vi "GPX_position_test.vi"() -> ()   [LabVIEW 2020]
panel:
  out "pos distance [m]":dbl
  out "acceleration graph":cluster{timestamp[], dbl[]}[](graph)
  out "gps mean speed":dbl format="%0.2f"
  out "distance [m]":dbl
  in  "shift [s]":dbl
  in  "Shift":bool
  out "delta t [s]":dbl
  in  "stop":bool
  in  "reset":bool
  in  "binary path (use dialog)":path
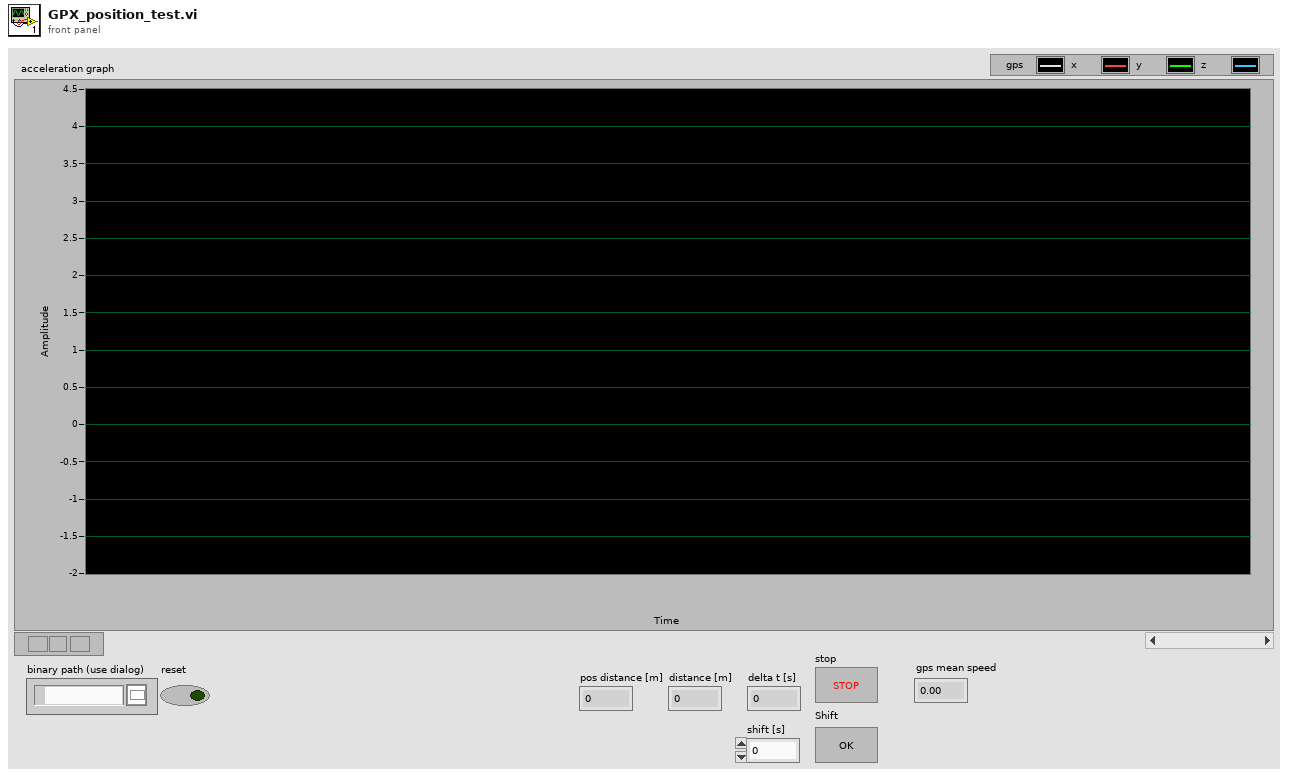
[diagram p1: front panel]
types:
  T1 = typedef "control_time_informations.ctl" = cluster{"starting time":timestamp, "ending time":timestamp, "dt[s]":dbl, "sampling rate [Hz]":dbl, "length":dbl}
  T2 = typedef "control_all_in_one_package.ctl" = cluster{"memory structure":T3, "actigraph settings":T4, "time informations":T1, "measurement data":T5}
  T3 = typedef "control_memory_structure.ctl" = cluster{"length of metadata [byte]":i32, "length of page [byte]":i32, "length of measurement data on page [byte]":i32, "length of dataset [byte]":i32}
  T4 = typedef "control_measurement_settings.ctl" = cluster{"sampling frequency [Hz]":dbl, "measurement interval [± g]":i32, "high precision?":bool, "number of pages":i32, "rate code":i32, "range code":i32, "id":i32}
  T5 = typedef "control_measurement_data.ctl" = cluster{"number of samples per axis":i32, "timestamp array":dbl[], "offset array":dbl[], "x, y, z axis data":waveform(dbl)[], "normalised magnitude of acceleartion vectors":waveform(dbl), "calibration coefficients":T6, "statistics":T7, "battery voltage":waveform(dbl), "magnitude of acceleartion vectors":waveform(dbl)}
  T6 = typedef "control_calibration_coefficients.ctl" = cluster{"Sx":dbl, "Ox":dbl, "Sy":dbl, "Oy":dbl, "Sz":dbl, "Oz":dbl}
  T7 = typedef "control_statistics.ctl" = cluster{"mean of x axis acceleration":dbl, "standard devation of x axis acceleration":dbl, "mean of y axis acceleration":dbl, "standard devation of y axis acceleration":dbl, "mean of z axis acceleration":dbl, "standard devation of z axis acceleration":dbl, "mean of normalised magnitude of acceleration":dbl, "standard devation of normalised magnitude of acceleration":dbl}
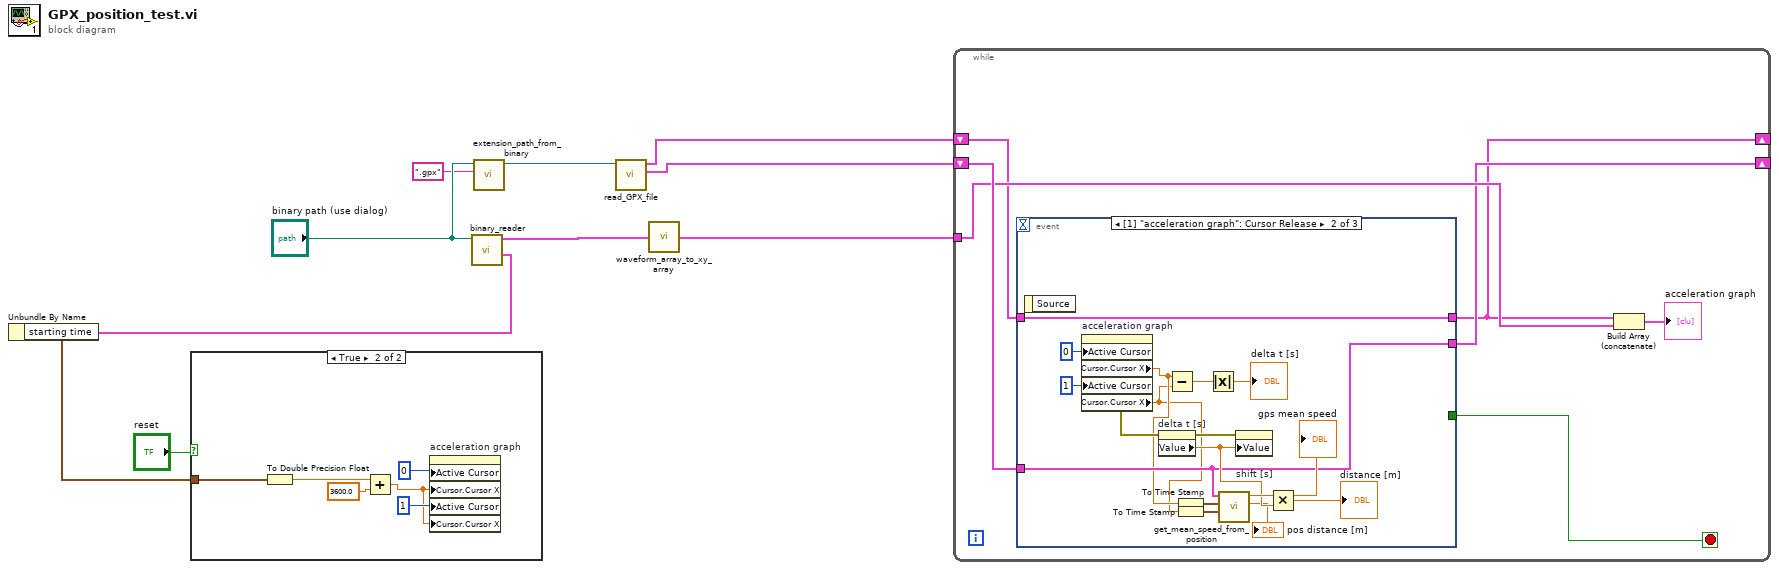
[diagram p0: block diagram]
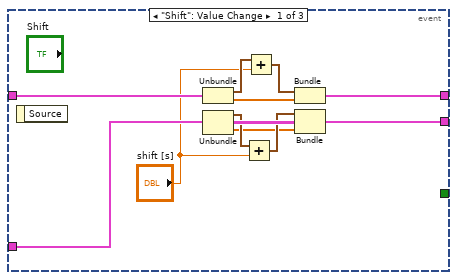
[diagram p2: hidden frame]
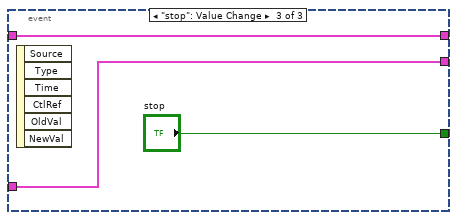
[diagram p3: hidden frame]
diagram:
  n1 = call "binary_reader.vi"("path to binary file"="binary path (use dialog)") -> ("time informations"=w9:T1, "all in one package"=w7:T2)  [unwired: 7 in, 1 out]
  n2 = Unbundle By Name(w9) -> ("starting time"=w8:timestamp)
  n3 = case shown="True" "reset" {
    tunnel: w8 -> [_ w14]
    frame False {
    }
    frame True {
      n4 = To Double Precision Float(number=w14) -> (double precision float=w15:dbl)
      n5 = Add(x=w15, y=3600.0) -> (x+y=w11:dbl)
      n6 = property on="acceleration graph" class="XYGraph (strict)"("Active Cursor"=u32 0, "Cursor.Cursor X"=w11, "Active Cursor"=u32 1, "Cursor.Cursor X"=w11) -> ()  [unwired: 2 in, 2 out]
    }
  }
  n7 = call "extension_path_from_binary.vi"("extension"=".gpx", "path to binary file"="binary path (use dialog)") -> ("path to file"=w2:path)  [unwired: 9 in]
  n8 = call "read_GPX_file.vi"("GPX File Path"=w2) -> ("lat/lon position"=w5:cluster{timestamp[], dbl[], dbl[]}, "XY Speed data"=w4:cluster{timestamp[], dbl[]})  [unwired: 3 in, 2 out]
  n9 = call "waveform_array_to_xy_array.vi"("waveform array"=w7) -> ("XY array"=w6:cluster{timestamp[], "Y":dbl[]}[])
  n10 = while {
    shift-right: [w19] -> _
    shift-left: w5 -> [w22]
    tunnel: w6 -> [w20]
    shift-right: [w17] -> _
    shift-left: w4 -> [w18]
    stop <- w23 stop-if-true
    n11 = event shown="[1] \"acceleration graph\": Cursor Release" {
      selector: _ -> [_ _ _]
      dyn-events: _ -> [_ _ _]
      timeout: _ -> [_ _ _]
      tunnel: [_ _ "stop"] -> w23
      tunnel: [w31 w42 w53] -> w19
      tunnel: w22 -> [w35 w42 w53]
      tunnel: w18 -> [w29 w37 w52]
      tunnel: [w24 w37 w52] -> w17
      event "Shift": Value Change {
        n12 = event-data() -> ()  [unwired: 1 in, 1 out]
        n13 = Unbundle(w29) -> (w28:timestamp[], w25:dbl[])
        n14 = Unbundle(w35) -> (w34:timestamp[], w32:dbl[], w30:dbl[])
        n15 = Add(x=w34, y="shift [s]") -> (x+y=w33:timestamp[])
        n16 = Add(x=w28, y="shift [s]") -> (x+y=w26:timestamp[])
        n17 = Bundle(w26, w25) -> (w24:cluster{timestamp[], dbl[]})  [unwired: 1 in]
        n18 = Bundle(w33, w32, w30) -> (w31:cluster{timestamp[], dbl[], dbl[]})  [unwired: 1 in]
      }
      event "acceleration graph": Cursor Release {
        n19 = event-data() -> ()  [unwired: 1 in, 1 out]
        n20 = property on="acceleration graph" class="XYGraph (strict)"("Active Cursor"=u32 0, "Active Cursor"=u32 1) -> (error out=w48:errorcluster, "Cursor.Cursor X"=w39:dbl, "Cursor.Cursor X"=w38:dbl)  [unwired: 2 in, 1 out]
        n21 = property on="delta t [s]" class="DigNum (strict)"(error in=w48) -> (error out=w47:errorcluster, "Value"=w44:dbl)  [unwired: 1 in, 1 out]
        n22 = Subtract(x=w39, y=w38) -> (x-y=w51:dbl)
        n23 = To Time Stamp(1:w39) -> (0:w40:timestamp)
        n24 = To Time Stamp(1:w38) -> (0:w41:timestamp)
        n25 = Absolute Value(x=w51) -> (abs(x)=→"delta t [s]":dbl)
        n26 = call "get_mean_speed_from_position.vi"("end"=w41, "start"=w40, "lat/lon position"=w42) -> ("distance [m]"=→"pos distance [m]":dbl, "mean speed [m/s]"=w46:dbl)  [unwired: 6 in, 1 out]
        "gps mean speed" <- w46
        n27 = property on="shift [s]" class="DigNum (strict)"(error in=w47, "Value"=w44) -> ()  [unwired: 1 in, 2 out]
        n28 = Multiply(x=w46, y=w44) -> (x*y=→"distance [m]":dbl)
      }
      event "stop": Value Change {
        n29 = event-data() -> ()  [unwired: 1 in, 6 out]
      }
    }
    n30 = Build Array (concatenate)(w17, w20) -> (→"acceleration graph":cluster{timestamp[], "Y":dbl[]}[])
  }
